vi "RunTestsCarWash.vi"() -> ()   [LabVIEW 2016]
uses:
  Drona.lvlib
  CarWashTest/CarWashTest.lvlib
panel:
  out "error out":errorcluster
  in  "Drona Tests PPL":path
  in  "EXE Path":path
  in  "Mode":string(combo)="Executable"
  # "*SourceCode - run from project instance"
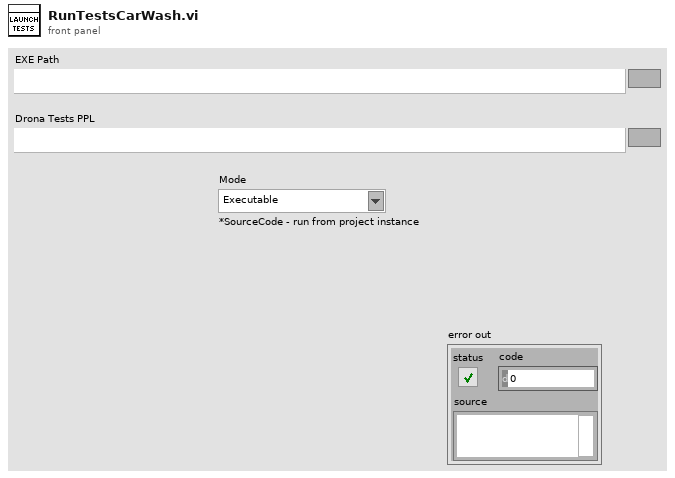
[diagram p1: front panel]
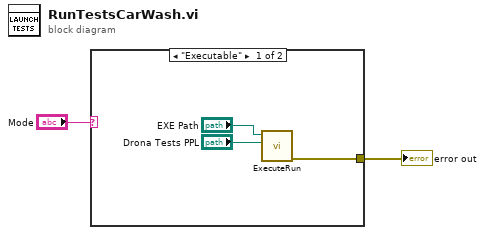
[diagram p0: block diagram]
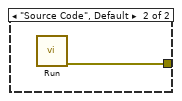
[diagram p2: hidden frame]
diagram:
  n1 = case shown="\"Executable\"" "Mode" {
    tunnel: [w3 w6] -> w1
    frame "Executable" {
      n2 = call "ExecuteRun.vi"("Drona Tests PPL"="Drona Tests PPL", "EXE Path"="EXE Path") -> ("error out"=w3:errorcluster)  [unwired: 9 in]
    }
    frame "Source Code", Default {
      n3 = call "Run.vi"() -> ("error out"=w6:errorcluster)  [unwired: 15 in]
    }
  }
  "error out" <- w1
